vi "Initialize.vi"(7 "Unload":bool, 8 "Error In":errorcluster, 11 "LabPack Shared Library In":path=path "") -> (0 "Error Out":errorcluster, 2 "Handle":u64, 3 "LabPack Shared Library Out":path)   [LabVIEW 2017, in "LabPack.lvlib" / "Writer.lvclass"]
uses:
  Writer.lvclass
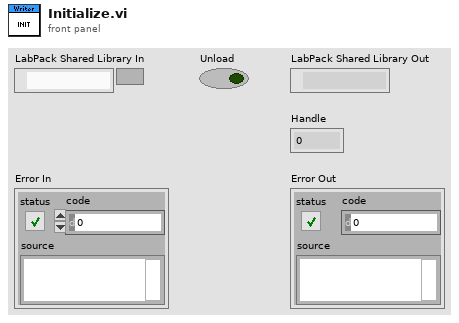
[diagram p1: front panel]
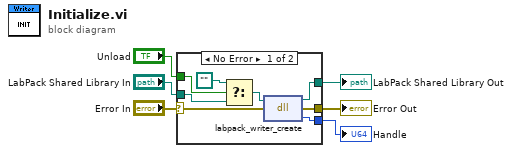
[diagram p0: block diagram]
diagram:
  n1 = case shown="No Error" "Error In" {
    selector: "Error In" -> [w7 w15]
    tunnel: "LabPack Shared Library In" -> [w13 _]
    tunnel: "Unload" -> [w11 _]
    tunnel: [w10 _] -> w4
    tunnel: [w9 w15] -> w3
    tunnel: [w8 _] -> w2
    frame No Error {
      n2 = Select(t=path "", s=w11, f=w13) -> (s? t:f=w14:path)
      n3 = dll-call lib="D:/Users/cfield/Code/MessagePack/LabPack/LabVIEW/trunk/src/LabPack/Private/labpack-x64.dll" fn="labpack_writer_create"(path in=w14, error in=w7) -> (path out=w8:path, error out=w9:errorcluster, "return type"=w10:u64)  [unwired: 1 in]
    }
    frame Error {
    }
  }
  "Handle" <- w4
  "Error Out" <- w3
  "LabPack Shared Library Out" <- w2
